vi "has_custom_lut_selected.vi"(8 "error in (no error)":errorcluster, 11 "DisplayDL090216 in":refnum<class "DisplayDL090216.lvclass">) -> (0 "error out":errorcluster, 1 "channel":refnum<vi>, 2 "has custom selected?":bool, 3 "DisplayDL090216 out":refnum<class "DisplayDL090216.lvclass">, 4 "index of element":i32)   [LabVIEW 2010, in "DisplayDL090216.lvclass"]
uses:
  DisplayDL090216.lvclass
  common/classes/Image/Image/colour_enum.ctl
  DisplayDL090216.lvclass/DisplayDL090216.ctl
  common/classes/Image/Image/Image.lvclass
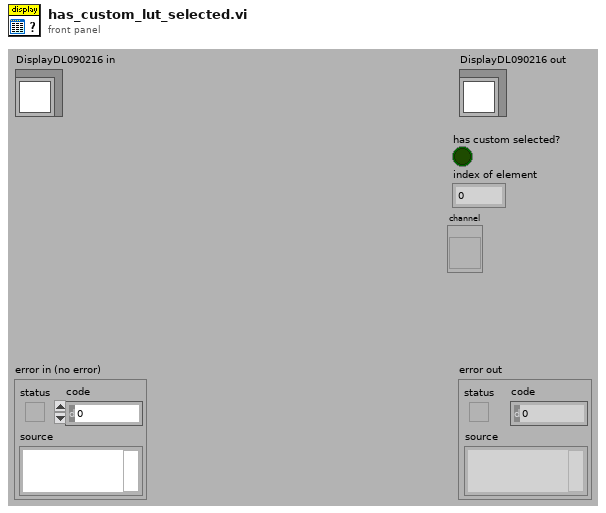
[diagram p1: front panel]
types:
  T1 = typedef "Image.lvclass/colour_enum.ctl" = enum16{"none", "red", "green", "blue", "grey scale", "custom"}
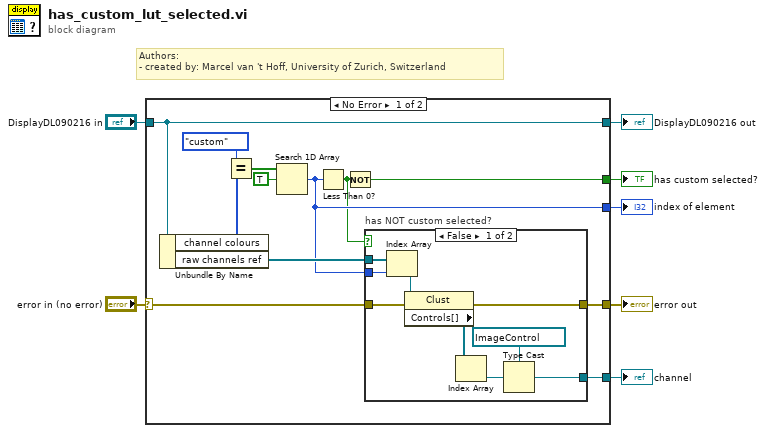
[diagram p0: block diagram]
diagram:
  # "Authors: \n- created by: Marcel van 't Hoff, University of Zurich, Switzerland"
  n1 = case shown="No Error" "error in (no error)" {
    selector: "error in (no error)" -> [w13 w31]
    tunnel: [w12 w31] -> w6
    tunnel: [w19 w30] -> w4
    tunnel: "DisplayDL090216 in" -> [w19 w30]
    tunnel: [w9 _] -> w2
    tunnel: [w14 _] -> w3
    tunnel: [w11 _] -> w1
    frame No Error {
      n2 = Unbundle By Name(w19) -> ("channel colours"=w15:T1[], "raw channels ref"=w10:refnum<vi>[])
      n3 = Equal?(x=colour_enum."custom" ("colour"), y=w15) -> (x = y?=w17:bool[])
      n4 = Search 1D Array(1D array=w17, element=TRUE) -> (index of element=w9:i32)  [unwired: 1 in]
      n5 = Less Than 0?(x=w9) -> (x < 0?=w8:bool)
      n6 = Not(x=w8) -> (.not. x?=w14:bool)
      n7 = case "has NOT custom selected?" shown="False" w8 {
        tunnel: w13 -> [w24 w29]
        tunnel: [w23 w29] -> w12
        tunnel: [w22 _] -> w11
        tunnel: w10 -> [w21 _]
        tunnel: w9 -> [w20 _]
        frame False {
          n8 = Index Array(array=w21, index=w20) -> (element=w25:refnum<vi>)
          n9 = property class="Clust"(reference=w25, error in=w24) -> (error out=w23:errorcluster, "Controls[]"=w26:refnum<vi>[])  [unwired: 1 out]
          n10 = Index Array(array=w26) -> (element=w27:refnum<vi>)  [unwired: 1 in]
          n11 = Type Cast(type=refnum<vi> refnum ("histogram out"), x=w27) -> (*(type *) &x=w22:refnum<vi>)
        }
        frame True {
        }
      }
    }
    frame Error {
    }
  }
  "error out" <- w6
  "DisplayDL090216 out" <- w4
  "has custom selected?" <- w3
  "index of element" <- w2
  "channel" <- w1
